vi "CAN Main2.vi"(8 "error in":errorcluster, 10 "Sequence Context In":refnum<k7>, 11 "Interface":refnum<k21>="CAN1") -> (0 "error out":errorcluster={"status"=TRUE, "code"=-1074384711, "source"="XNET Create Session (Signal Input Single-point).vi:6590002<APPEND>\n\n<b>Complete call chain:</b>\r\n     XNET Create Session (Signal Input Single-point).vi:6590002\r\n     CAN GIP.lvlib:GIP CAN Wrapper.vi:2150001\r\n     CAN GIP.lvlib:CAN GIP Test.vi"})   [LabVIEW 2021, in "CAN wrapper.lvlib"]
uses:
  CAN wrapper.lvlib
  Private Controls/CAN States.ctl
  Private Controls/Setting.ctl
  <vilib>/addons/TestStand/_TSUtility.llb/TestStand - Get Property Value (String).vi
  <vilib>/addons/TestStand/_TSUtility.llb/TestStand - Get Property Value (Boolean).vi
  <vilib>/addons/TestStand/_TSUtility.llb/TestStand - Get Property Value (Number).vi
  <vilib>/addons/TestStand/_TSUtility.llb/TestStand - Set Property Value (Number).vi
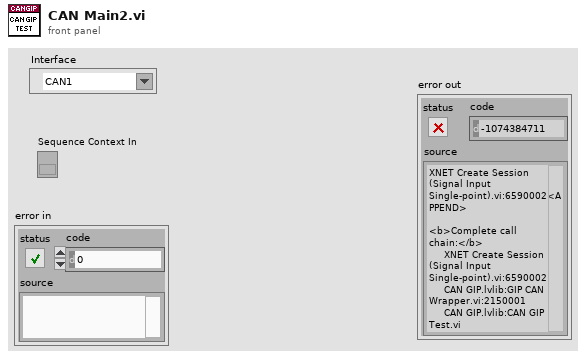
[diagram p1: front panel]
types:
  T1 = typedef "CAN wrapper.lvlib/CAN States.ctl" = enum16{"Init", "Config", "Read Signals", "Write Signals", "Close"}
  T2 = typedef "CAN wrapper.lvlib/Setting.ctl" = cluster{"Termination":u32, "Baud Rate":u64, "Interface":refnum<k21>, "XNET Database":refnum<k21>, "ECU":refnum<k21>}
  T3 = typedef "TestStand - Status Monitor.ctl" = cluster{"Sequence Context":refnum<k7>, "Execution":refnum<k7>, "Termination Monitor":refnum<k7>}
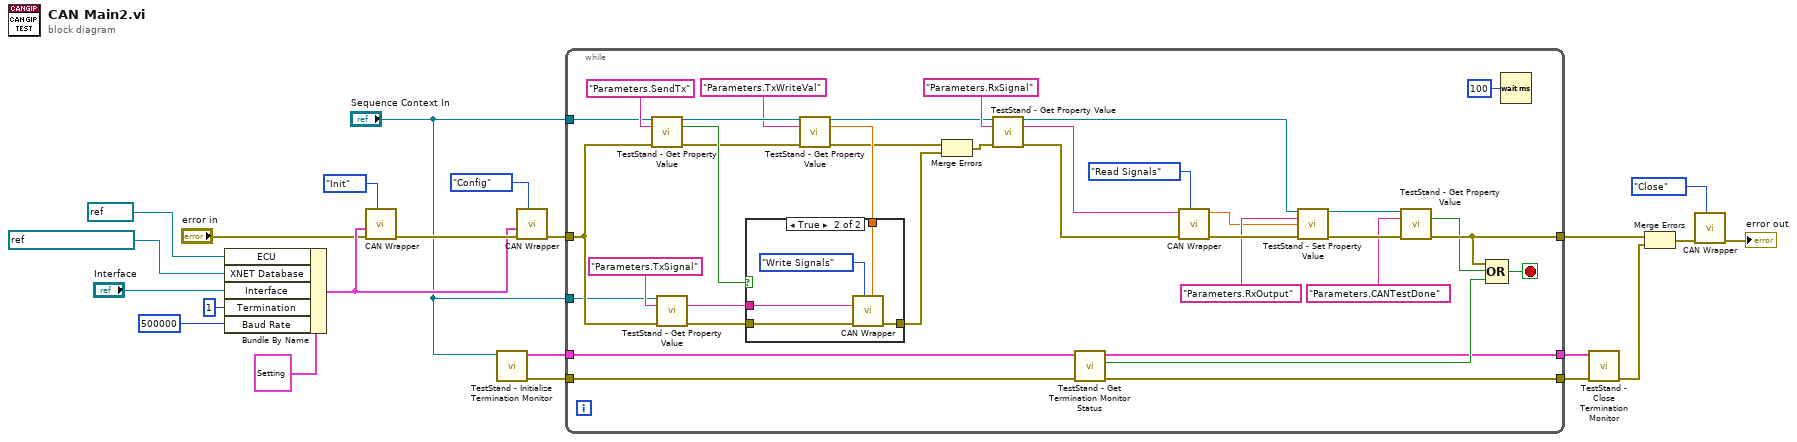
[diagram p0: block diagram]
diagram:
  n1 = Bundle By Name(cluster=T2 {"Termination"=1, "Baud Rate"=125000, "Interface"="CAN1", "XNET Database"="GIP_CAN_Database", "ECU"="GIP\nGIP_CAN_Database"} ("Setting"), "ECU"=refnum<k21> "GIP\ncan_messages_818", "XNET Database"=refnum<k21> "can_messages_818", "Interface"="Interface", "Termination"=u32 1, "Baud Rate"=u64 500000) -> (w18:T2)
  n2 = call "CAN Wrapper.vi"("States"=CAN_States."Init" ("CAN States"), "error in"="error in", "Setting"=w18) -> ("error out"=w21:errorcluster)  [unwired: 7 in, 1 out]
  n3 = call <vilib>:"TestStand - Initialize Termination Monitor.vi"("Sequence Context In"="Sequence Context In") -> ("error out"=w10:errorcluster, "Status Monitor Out"=w9:T3)  [unwired: 9 in]
  n4 = call "CAN Wrapper.vi"("States"=CAN_States."Config" ("CAN States"), "error in"=w21, "Setting"=w18) -> ("error out"=w17:errorcluster)  [unwired: 7 in, 1 out]
  n5 = while {
    tunnel: [w41] -> w6
    tunnel: w17 -> [w35]
    tunnel: w10 -> [w58]
    tunnel: "Sequence Context In" -> [w37]
    tunnel: w9 -> [w57]
    tunnel: [w54] -> w7
    tunnel: [w53] -> w8
    tunnel: "Sequence Context In" -> [w34]
    stop <- w56 stop-if-true
    n6 = call-poly <vilib>:"TestStand - Get Property Value.vi"("Sequence Context In"=w37, "Lookup String"="Parameters.SendTx", "error in (no error)"=w35) -> ("Sequence Context Out"=w32:refnum<k7>, "Value"=w31:bool, "error out"=w30:errorcluster)  [unwired: 10 in]
    n7 = call-poly <vilib>:"TestStand - Get Property Value.vi"("Sequence Context In"=w34, "Lookup String"="Parameters.TxSignal", "error in (no error)"=w35) -> ("Value"=w33:string, "error out"=w28:errorcluster)  [unwired: 10 in, 1 out]
    n8 = call-poly <vilib>:"TestStand - Get Property Value.vi"("Sequence Context In"=w32, "Lookup String"="Parameters.TxWriteVal", "error in (no error)"=w30) -> ("Sequence Context Out"=w26:refnum<k7>, "Value"=w27:dbl, "error out"=w25:errorcluster)  [unwired: 10 in]
    n9 = case shown="True" w31 {
      tunnel: w33 -> [_ w61]
      tunnel: w28 -> [w59 w63]
      tunnel: w27 -> [_ w62]
      tunnel: [w59 w60] -> w24
      frame False {
      }
      frame True {
        n10 = call "CAN Wrapper.vi"("Signal Write"=w62, "States"=CAN_States."Write Signals" ("CAN States"), "error in"=w63, "Tx Signal In"=w61) -> ("error out"=w60:errorcluster)  [unwired: 6 in, 1 out]
      }
    }
    n11 = Merge Errors(w25, w24) -> (w23:errorcluster)
    n12 = call-poly <vilib>:"TestStand - Get Property Value.vi"("Sequence Context In"=w26, "Lookup String"="Parameters.RxSignal", "error in (no error)"=w23) -> ("Sequence Context Out"=w45:refnum<k7>, "Value"=w49:string, "error out"=w51:errorcluster)  [unwired: 10 in]
    n13 = call <vilib>:"TestStand - Get Termination Monitor Status.vi"("error in (no error)"=w58, "Status Monitor In"=w57) -> ("error out"=w54:errorcluster, "Terminating or Aborting"=w55:bool, "Status Monitor Out"=w53:T3)  [unwired: 7 in]
    n14 = call "CAN Wrapper.vi"("States"=CAN_States."Read Signals" ("CAN States"), "error in"=w51, "Rx Signal In"=w49) -> ("error out"=w46:errorcluster, "Signal out"=w43:dbl)  [unwired: 7 in]
    n15 = call-poly <vilib>:"TestStand - Set Property Value.vi"("Sequence Context In"=w45, "Lookup String"="Parameters.RxOutput", "New Value"=w43, "error in (no error)"=w46) -> ("Sequence Context Out"=w40:refnum<k7>, "error out"=w42:errorcluster)  [unwired: 10 in]
    n16 = call-poly <vilib>:"TestStand - Get Property Value.vi"("Sequence Context In"=w40, "Lookup String"="Parameters.CANTestDone", "error in (no error)"=w42) -> ("Value"=w38:bool, "error out"=w41:errorcluster)  [unwired: 10 in, 1 out]
    n17 = Compound Arithmetic op=OR(w41, w38, w55) -> (w56:bool)
    n18 = Wait (ms)(milliseconds to wait=u32 100) -> ()  [unwired: 1 out]
  }
  n19 = call <vilib>:"TestStand - Close Termination Monitor.vi"("error in (no error)"=w7, "Status Monitor In"=w8) -> ("error out"=w5:errorcluster)  [unwired: 9 in]
  n20 = Merge Errors(w6, w5) -> (w3:errorcluster)
  n21 = call "CAN Wrapper.vi"("States"=CAN_States."Close" ("CAN States"), "error in"=w3) -> ("error out"=→"error out":errorcluster)  [unwired: 8 in, 1 out]
